vi "NI VeriStand - Set Custom Device Channel Value Table_offline.vi"(8 "error in (no error)":errorcluster, 9 "Values":dbl[](array[numeric]), 10 "Names":string[](array[string]), 11 "Channel Ref in":T1 format="%.0x") -> (0 "error out":errorcluster, 3 "Channel Ref out":T1=18446744073709551615 format="%.0x")   [LabVIEW 2020, in "AIM MIL-STD 1553 Shared.lvlib"]
uses:
  <vilib>/NI VeriStand/Custom Device API/Custom Device Item Ref.ctl
  NationalInstruments.VeriStand.SystemDefinitionAPI
  NationalInstruments.VeriStand.SystemStorage
  AIM MIL-STD 1553 Shared.lvlib
  <vilib>/NI VeriStand/Custom Device API/Custom Device API.lvlib
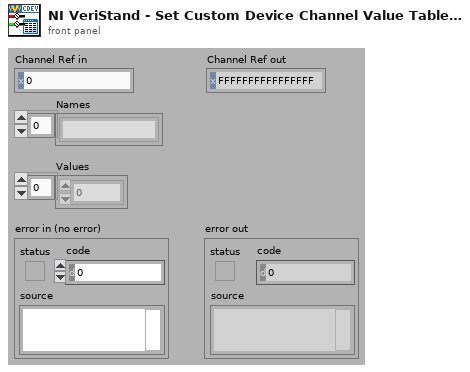
[diagram p1: front panel]
types:
  T1 = typedef "Custom Device API.lvlib/Custom Device Item Ref.ctl" = u64
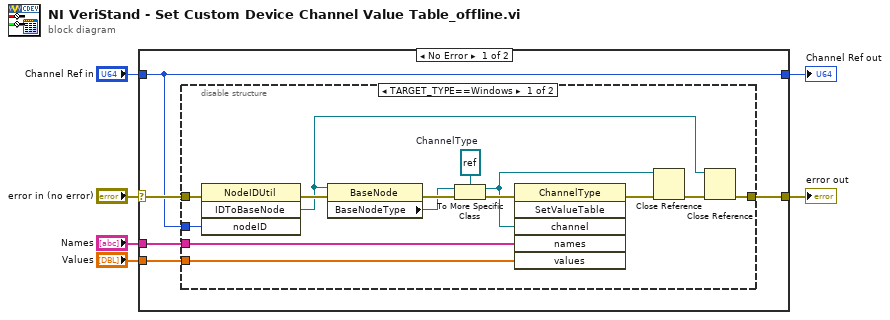
[diagram p0: block diagram]
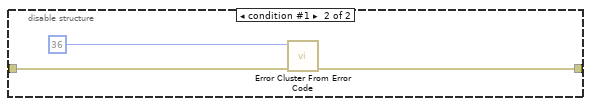
[diagram p2: hidden frame]
diagram:
  n1 = case shown="No Error" "error in (no error)" {
    selector: "error in (no error)" -> [w11 w30]
    tunnel: [w9 w30] -> w6
    tunnel: "Channel Ref in" -> [w10 w29]
    tunnel: [w10 w29] -> w4
    tunnel: "Names" -> [w8 _]
    tunnel: "Values" -> [w7 _]
    frame No Error {
      n2 = disable-structure shown="TARGET_TYPE==Windows" {
        disable-tunnel: w11 -> [w19 w28]
        disable-tunnel: w10 -> [w18 _]
        disable-tunnel: [w13 w27] -> w9
        disable-tunnel: w8 -> [w21 _]
        disable-tunnel: w7 -> [w22 _]
        frame condition #0 (active) {
          w23 = refnum<k24> refnum  # ChannelType
          n3 = invoke class="NodeIDUtil" method="IDToBaseNode"(error in=w19, "nodeID"=w18) -> (error out=w17:errorcluster, "IDToBaseNode"=w12:refnum<k24>)  [unwired: 2 in, 2 out]
          n4 = property class="BaseNode"(reference=w12, error in=w17) -> (error out=w16:errorcluster, "BaseNodeType"=w15:refnum<k24>)  [unwired: 1 out]
          n5 = To More Specific Class(target class=w23, reference=w15, error in=w16) -> (specific class reference=w20:refnum<k24>, error out=w25:errorcluster)
          n6 = invoke class="ChannelType" method="SetValueTable"(error in=w25, "channel"=w20, "names"=w21, "values"=w22) -> (error out=w24:errorcluster)  [unwired: 2 in, 5 out]
          n7 = Close Reference(reference=w20, error in (no error)=w24) -> (error out=w14:errorcluster)
          n8 = Close Reference(reference=w12, error in (no error)=w14) -> (error out=w13:errorcluster)
        }
        frame condition #1 {
          n9 = call <vilib>:"Error Cluster From Error Code.vi"("error in (no error)"=w28, "error code (0)"=36) -> ("error out"=w27:errorcluster)  [unwired: 7 in]
        }
      }
    }
    frame Error {
    }
  }
  "error out" <- w6
  "Channel Ref out" <- w4
